vi "Write angExp.vi"(8 "error in":errorcluster, 10 "angExp":sgl, 11 "cPAS Data in":refnum<class "cPAS Data.lvclass">) -> (0 "error out":errorcluster, 3 "cPAS Data out":refnum<class "cPAS Data.lvclass">)   [LabVIEW 2015, in "cPAS Data.lvclass"]
doc: "Write the Angstrom exponent to the cPAS data class."
uses:
  cPAS Data.lvclass
  cPAS Data.lvclass/cPAS Data.ctl
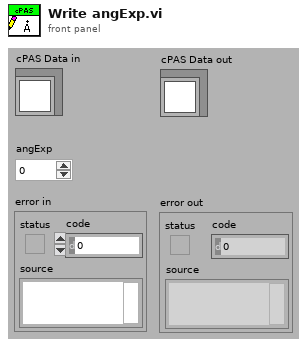
[diagram p1: front panel]
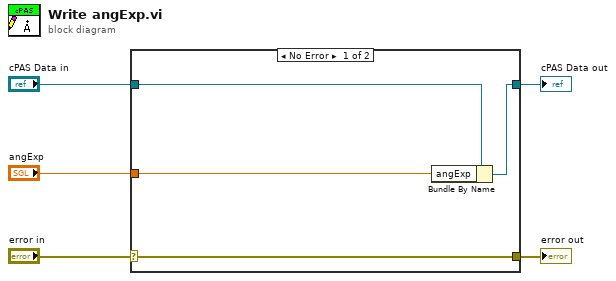
[diagram p0: block diagram]
diagram:
  n1 = case shown="No Error" "error in" {
    selector: "error in" -> [w9 w10]
    tunnel: [w9 w10] -> w4
    tunnel: [w7 w11] -> w2
    tunnel: "cPAS Data in" -> [w8 w11]
    tunnel: "angExp" -> [w6 _]
    frame No Error {
      n2 = Bundle By Name(cluster=w8, "angExp"=w6) -> (w7:refnum<class "cPAS Data.lvclass">)
    }
    frame Error {
    }
  }
  "error out" <- w4
  "cPAS Data out" <- w2
